vi "Init Msg Output.vi"() -> (3 "Stopping Msg Output out":refnum<class "Stopping Msg Output.lvclass">)   [LabVIEW 2020, in "jettl.lvlib" / "Stopping jettl Msg.lvlib" / "Stopping Msg Output.lvlib" / "Stopping Msg Output.lvclass"]
doc: "jettl 6.12.1.94\nNathan Davis - Nathan Davis\nCopyright (c) 2026, Nathan Davis\nMIT"
uses:
  Stopping Msg Output.lvclass
  Stopping Msg Output.lvclass/Stopping Msg Output.ctl
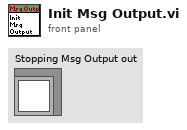
[diagram p1: front panel]
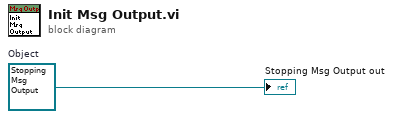
[diagram p0: block diagram]
diagram:
  w1 = refnum<class "Stopping Msg Output.lvclass"> refnum  # Object
  "Stopping Msg Output out" <- w1
